vi "RT_Propulsive_Moment_in_DLR_Navigation_Reference_System(SubVI).vi"(5 "FE":dbl[](array[numeric]), 7 "le (m) in":dbl, 9 "DCM":dbl[][](array[numeric]), 10 "i":i32, 11 "Data":dbl[][](array[numeric])) -> (3 "MFE (Nm)":dbl[](array[numeric]))   [LabVIEW 2017]
uses:
  <vilib>/Analysis/baseanly.llb/Real A x B.vi
  <vilib>/Analysis/Matrix/Numeric/Conversions/Array To Matrix - RA2.vi
  <vilib>/Analysis/Matrix/Numeric/Conversions/Array To Matrix - RA.vi
  <vilib>/Analysis/Matrix/Numeric/Conversions/Matrix To Array - RM.vi
  <vilib>/Analysis/NI_AALBase.lvlib
  <vilib>/Analysis/Matrix/NI_Matrix.lvlib
  <vilib>/Analysis/NI_AALPro.lvlib
panel:
  out "Re":dbl[](array[numeric])
  out "re":dbl
  out "CoG (m)":dbl
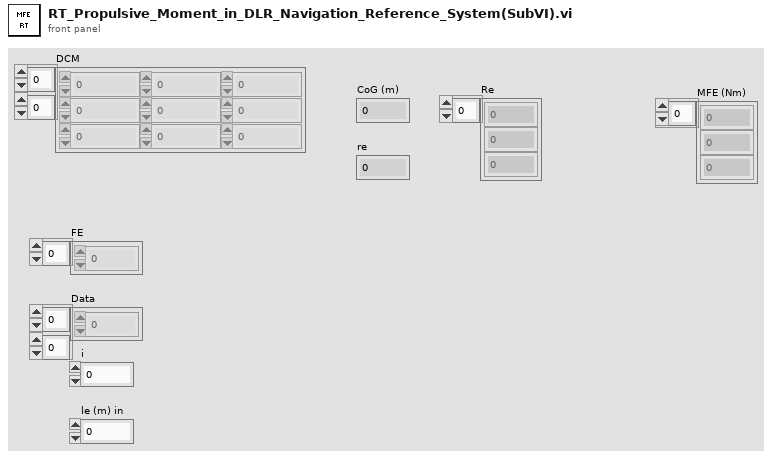
[diagram p1: front panel]
types:
  T1 = typedef "NI_Matrix.lvlib/RealMatrix.ctl" = dbl[][]
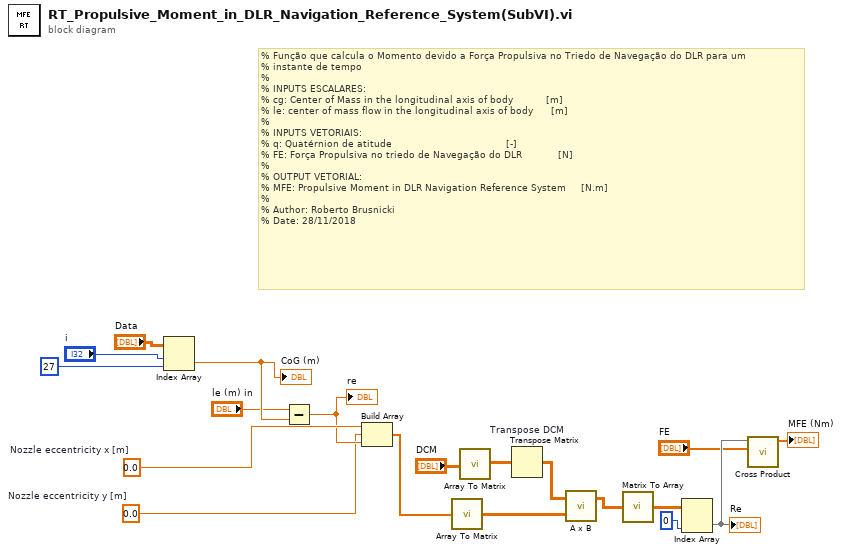
[diagram p0: block diagram]
diagram:
  w1 = 0.0  # Nozzle eccentricity y [m]
  w11 = 0.0  # Nozzle eccentricity x [m]
  # "% Função que calcula o Momento devido a Força Propulsiva no Triedo de Navegação do DLR para um \n% instante de tempo\n%\n% INPUTS ESCALARES:\n% cg: Center of Mass in the longitudinal axis of body           [m]\n% le: center of mass flow in the longitudinal axis of body      [m]\n% \n% INPUTS VETORIAIS:\n% q: Quatérnion de atitude                                      [-]\n% FE: Força Propulsiva no triedo de Navegação do DLR            [N] \t\n%\n% OUTPUT VETORIAL:\n% MFE: Propulsive Moment in DLR Navigation Reference System     [N.m]\n%\n% Author: Roberto Brusnicki\n% Date: 28/11/2018"
  n1 = Index Array(array="Data", index (row)="i", index (col)=27 ("disabled index (col)")) -> (element=w16:dbl)
  "CoG (m)" <- w16
  n2 = Subtract(x="le (m) in", y=w16) -> (x-y=w10:dbl)
  "re" <- w10
  n3 = Build Array(w11, w1, w10) -> (w12:dbl[])
  n4 = call-poly <vilib>:"Array To Matrix.vi"("Real 1D Array"=w12) -> ("Real Matrix (Column Vector)"=w9:T1)
  n5 = call-poly <vilib>:"Array To Matrix.vi"("Real 2D Array"="DCM") -> ("Real Matrix"=w13:T1)
  n6 = Transpose Matrix "Transpose DCM"(1:w13) -> (0:w14:T1)
  n7 = call-poly <vilib>:"A x B.vi"("B"=w9, "A"=w14) -> ("A x B"=w7:T1)  [unwired: 1 out]
  n8 = call-poly <vilib>:"Matrix To Array.vi"("Real Matrix"=w7) -> ("Real 2D Array"=w8:dbl[][])
  n9 = Index Array(array=w8, index (col)=0 ("index (row)")) -> (element=w18:dbl[])  [unwired: 1 in]
  "Re" <- w18
  n10 = call <vilib>:"Cross Product.vi"("B Vector"="FE", "A Vector"=w18) -> ("Cross Product"=→"MFE (Nm)":dbl[])  [unwired: 8 in, 1 out]
